vi "强制类型转换DBL to I64.vi"() -> ()   [LabVIEW 2020]
doc: "本VI是为《我和LabVIEW》一书编写的示例。\n关于本书的介绍请参考网页：\nhttp://ruanqizhen.spaces.live.com/blog/cns!5852D4F797C53FB6!4310.entry"
panel:
  out "64位整型":i64
  out "I64数据":i64 format="%.0b"
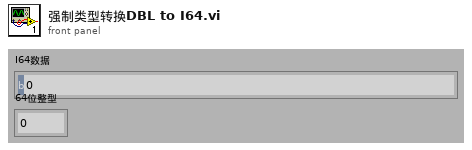
[diagram p1: front panel]
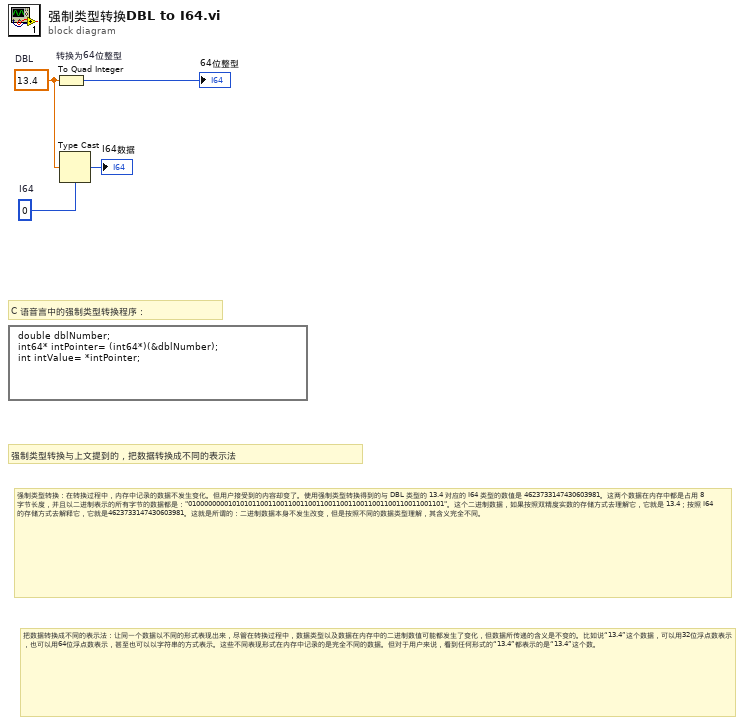
[diagram p0: block diagram]
diagram:
  w4 = i64 0  # I64
  w1 = 13.4  # DBL
  # "把数据转换成不同的表示法：让同一个数据以不同的形式表现出来，尽管在转换过程中，数据类型以及数据在内存中的二进制数值可能都发生了变化，但数据所传递的含义是不变的。比如说“13.4”这个数据，可以用32位浮点数表示，也可以用64位浮点数表示，甚至也可以以字符串的方式表示。这些不同表现形式在内存中记录的是完全不同的数据。但对于用户来说，看到任何形式的“13.4”都表示的是“13.4”这个数。"
  # "强制类型转换：在转换过程中，内存中记录的数据不发生变化。但用户接受到的内容却变了。使用强制类型转换得到的与 DBL 类型的 13.4 对应的 I64 类型的数值是 4623733147430603981。这两个数据在内存中都是占用 8 字节长度，并且以二进制表示的所有字节的数据都是：\"0100000000101010110011001100110011001100110011001100110011001101\"。这个二进制数据，如果按照双精度实数的存储方式去理解它，它就是 13.4；按照 I64 的存储方式去解释它，它就是4623733147430603981。这就是所谓的：二进制数据本身不发生改变，但是按照不同的数据类型理解，其含义完全不同。"
  # "强制类型转换与上文提到的，把数据转换成不同的表示法"
  # "C 语音言中的强制类型转换程序："
  n1 = formula code="double dblNumber;\nint64* intPointer= (int64*)(&dblNumber);\nint intValue= *intPointer;"() -> ()
  n2 = To Quad Integer "转换为64位整型"(1:w1) -> (0:→"64位整型":i64)
  n3 = Type Cast ("强制类型转换")(type=w4, x=w1) -> (*(type *) &x=→"I64数据":i64)
